vi "_Persist New Entity.vi"(8 "error in (no error)":errorcluster, 10 "New Entity":refnum<class "Entity.lvclass">, 11 "Entity Manager in":refnum<class "Entity Manager.lvclass">) -> (0 "error out":errorcluster, 2 "Entity ID":T1, 3 "Entity Manager out":refnum<class "Entity Manager.lvclass">)   [LabVIEW 2020, in "Conditu2.lvlib" / "Entity Manager.lvclass"]
uses:
  Entity Manager.lvclass
  Entity/Entity.lvclass
  Entity ID.ctl
  Entity Manager.lvclass/Entity Manager.ctl
  Database Platform/Database Platform.lvclass
  Conditu2.lvlib
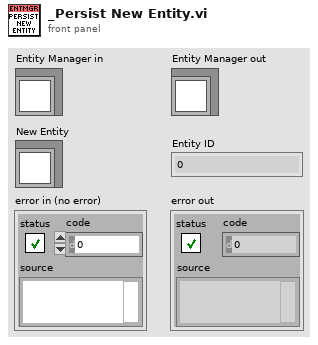
[diagram p1: front panel]
types:
  T1 = typedef "Conditu2.lvlib/Entity ID.ctl" = i64
  T2 = typedef "Conditu2.lvlib/Entity Manager.lvclass/Known Entity.ctl" = cluster{"Entity":refnum<class "Entity.lvclass">, "Types":refnum<class "Type.lvclass">[], "Type Name Map":map{string, i32}}
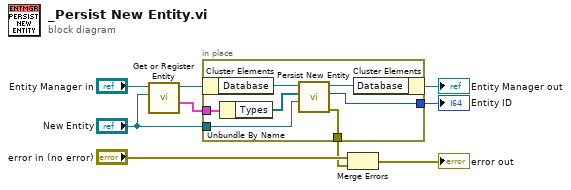
[diagram p0: block diagram]
diagram:
  n1 = call "Get or Register Entity.vi"("Entity"="New Entity", "Entity Manager in"="Entity Manager in") -> ("Entity Info"=w1:T2, "Entity Manager out"=w3:refnum<class "Entity Manager.lvclass">)  [unwired: 8 in]
  n2 = in-place {
    in-place-border: "New Entity" -> [w12]
    in-place-border: [w14] -> w8
    in-place-border: [w13] -> w5
    in-place-border: w1 -> [w11]
    n3 = in-place-cluster #1(w3) -> ("Database"=w16:refnum<class "Database Platform.lvclass">)
    n4 = Unbundle By Name(w11) -> ("Types"=w10:refnum<class "Type.lvclass">[])
    n5 = call-dynamic "Persist New Entity.vi"("Entity"=w12, "Types"=w10, "Database in"=w16) -> ("error out"=w13:errorcluster, "New ID"=w14:T1, "Database out"=w15:refnum<class "Database Platform.lvclass">)  [unwired: 6 in]
    n6 = in-place-cluster #1("Database"=w15) -> (→"Entity Manager out":refnum<class "Entity Manager.lvclass">)
  }
  "Entity ID" <- w8
  n7 = Merge Errors("error in (no error)", w5) -> (→"error out":errorcluster)
